vi "Gain Offset.vi"(11 "Values Read":dbl[](array[numeric])) -> (3 "Dynamic Data Type":dynamicdata(waveform))   [LabVIEW 2019]
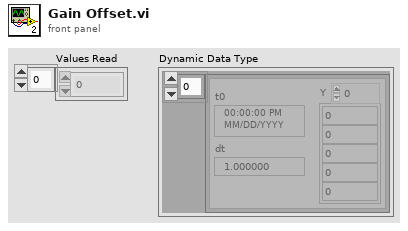
[diagram p1: front panel]
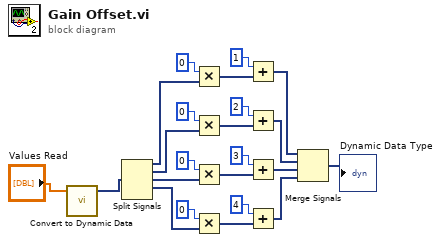
[diagram p0: block diagram]
diagram:
  n1 = call "Convert to Dynamic Data"("Array"="Values Read") -> ("Dynamic Data Type"=w22:dynamicdata)  [unwired: 3 in]
  n2 = Split Signals(w22) -> (w20:dynamicdata, w12:dynamicdata, w7:dynamicdata, w2:dynamicdata)  [unwired: 5 in, 1 out]
  n3 = Multiply(x=0, y=w20) -> (x*y=w19:dynamicdata)
  n4 = Multiply(x=0, y=w12) -> (x*y=w15:dynamicdata)
  n5 = Multiply(x=0, y=w7) -> (x*y=w10:dynamicdata)
  n6 = Multiply(x=0, y=w2) -> (x*y=w5:dynamicdata)
  n7 = Add(x=1, y=w19) -> (x+y=w18:dynamicdata)
  n8 = Add(x=2, y=w15) -> (x+y=w11:dynamicdata)
  n9 = Add(x=3, y=w10) -> (x+y=w6:dynamicdata)
  n10 = Add(x=4, y=w5) -> (x+y=w1:dynamicdata)
  n11 = Merge Signals(w18, w11, w6, w1) -> (→"Dynamic Data Type":dynamicdata)
